vi "getReference.vi"(8 "error in (no error)":errorcluster, 11 "TransactionListUserInterface in":refnum<class "TransactionListUIAdapter.lvclass">) -> (0 "error out":errorcluster, 2 "MulticolumnListbox":refnum<vi>, 3 "TransactionListUserInterface out":refnum<class "TransactionListUIAdapter.lvclass">)   [LabVIEW 2018, in "TransactionListUIAdapter.lvclass"]
uses:
  TransactionListUIAdapter.lvclass
  TransactionListUIAdapter.lvclass/TransactionListUIAdapter.ctl
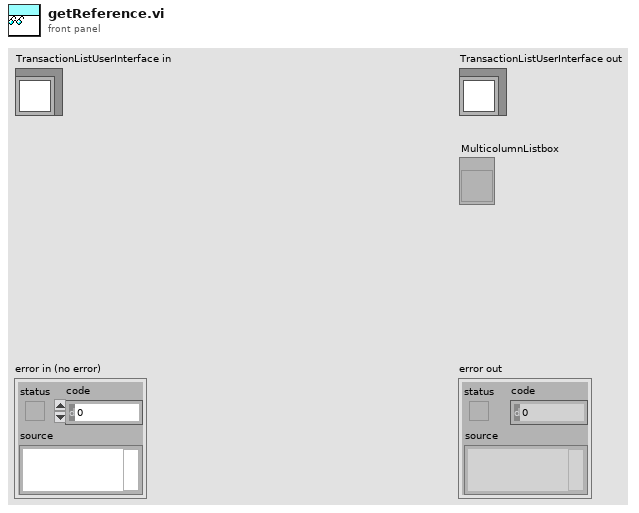
[diagram p1: front panel]
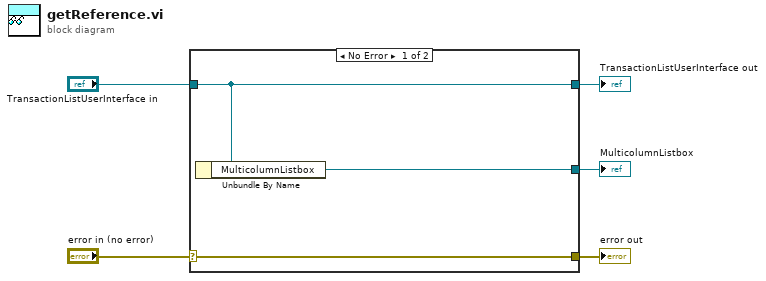
[diagram p0: block diagram]
diagram:
  n1 = case shown="No Error" "error in (no error)" {
    selector: "error in (no error)" -> [w8 w9]
    tunnel: [w8 w9] -> w4
    tunnel: [w7 w10] -> w2
    tunnel: "TransactionListUserInterface in" -> [w7 w10]
    tunnel: [w6 _] -> w1
    frame No Error {
      n2 = Unbundle By Name(w7) -> ("MulticolumnListbox"=w6:refnum<vi>)
    }
    frame Error {
    }
  }
  "error out" <- w4
  "TransactionListUserInterface out" <- w2
  "MulticolumnListbox" <- w1
